vi "NewPathAvailCheck.vi"() -> (3 "New Path Available":bool)   [LabVIEW 2019]
uses:
  <vilib>/Rock Robotics/WPI/ThirdParty/MJansen/PathPlanner/VI/PathPlanner_PathFinder_Globals.vi
  <vilib>/Rock Robotics/WPI/ThirdParty/MJansen/PathPlanner/PathPlanner24.lvlib
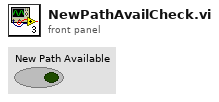
[diagram p1: front panel]
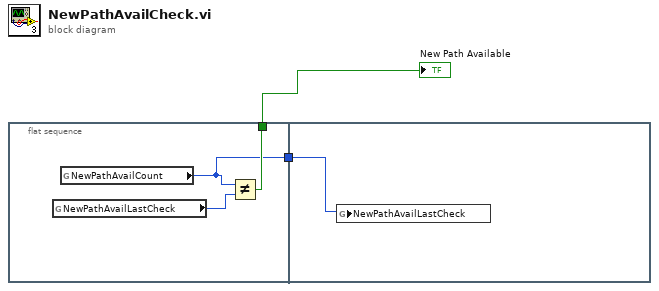
[diagram p0: block diagram]
diagram:
  n1 = flat-sequence {
    tunnel: [w4] -> w2
    tunnel: [w3] -> w1
    tunnel: w1 -> [w6]
    frame #0 {
      n2 = global read "PathPlanner_PathFinder_Globals.vi" "NewPathAvailLastCheck"() -> (w5:i32)
      n3 = global read "PathPlanner_PathFinder_Globals.vi" "NewPathAvailCount"() -> (w3:i32)
      n4 = Not Equal?(x=w3, y=w5) -> (x != y?=w4:bool)
    }
    frame #1 {
      n5 = global write "PathPlanner_PathFinder_Globals.vi" "NewPathAvailLastCheck"(w6) -> ()
    }
  }
  "New Path Available" <- w2
